vi "Destroy.vi"   [LabVIEW 2018, in "Toolkit.lvlib" / "Known Host.lvclass"]
doc: "Destroys this Known Host object and frees the memory allocated for the libssh2lv shared library Known Host struct. No other VIs should be executed after this VI has completed."
uses:
  Known Host.lvclass
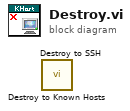
[diagram p0: block diagram]
diagram:
  n1 = call "Destroy to Known Hosts.vi"() -> ()  [unwired: 10 in, 2 out]
  n2 = call "Destroy to SSH.vi"() -> ()  [unwired: 10 in, 2 out]
